vi "Shoot.vi"(3 "Shooter Position (0 to 8)":i8(slide) scale=0.0..4.0) -> (0 "Inside Perimeter":bool=TRUE, 1 "In Position":bool=TRUE)   [LabVIEW 2012]
uses:
  Robot Global Data.vi
  <vilib>/Rock Robotics/WPI/Joystick/WPI_JoystickGetSetRefNum.vi
panel:
  out "Joystick Override":bool=TRUE
  in  "Inbound OLD RBT":dbl=1.7
  in  "Inbound NEW RBT":dbl=1.7
  in  "Upper Perimeter OLD":dbl=0.1
  in  "Lower Perimeter OLD":dbl=3.4
  in  "Rest OLD RBT":dbl=2.5
  in  "Load OLD RBT":dbl=2.5
  in  "Shoot OLD RBT":dbl=1.5
  in  "PID gains\nOLD RBT":T1={"proportional gain (Kc)"=0.5, "integral time (Ti, min)"=0.0, "derivative time (Td, min)"=0.0} {"derivative time (Td, min)" format="%.3f"; "integral time (Ti, min)" format="%.3f"; "proportional gain (Kc)" format="%.3f"}
  in  "Max Speeds\nOLD RBT":cluster{"Down Speed":dbl, "Up Speed":dbl}={"Down Speed"=0.3, "Up Speed"=-0.3} {"Up Speed" format="%.2f"; "Down Speed" format="%.2f"}
  in  "PID gains\nNEW RBT":T1={"proportional gain (Kc)"=0.5, "integral time (Ti, min)"=0.0, "derivative time (Td, min)"=0.0} {"derivative time (Td, min)" format="%.3f"; "integral time (Ti, min)" format="%.3f"; "proportional gain (Kc)" format="%.3f"}
  in  "Max Speeds\nNEW RBT":cluster{"Down Speed":dbl, "Up Speed":dbl}={"Down Speed"=0.2, "Up Speed"=-0.35} {"Up Speed" format="%.2f"; "Down Speed" format="%.2f"}
  in  "Upper Perimeter NEW":dbl=3.8
  in  "Lower Perimeter NEW":dbl=0.6
  in  "Dead Zone":dbl=0.1
  in  "Rest NEW RBT":dbl=4.0
  in  "Load NEW RBT":dbl=0.5
  in  "Shoot NEW RBT":dbl=1.9
  out "output":dbl=0.04258389399999998
  out "Pot Voltage":dbl=0.41483221200000003
  # "OLD"
  # "NEW"
  # "0.5"
  # "0.5"
  # "0.2"
  # "0.3"
  # "0"
  # "0"
  # "-.35"
  # "-0.3"
  # "New"
  # "3"
  # "1.9"
  # "0.6"
  # "2.5"
  # "0.5"
  # "3.8"
  # "2.5"
  # "4"
  # "1.7"
  # "1.7"
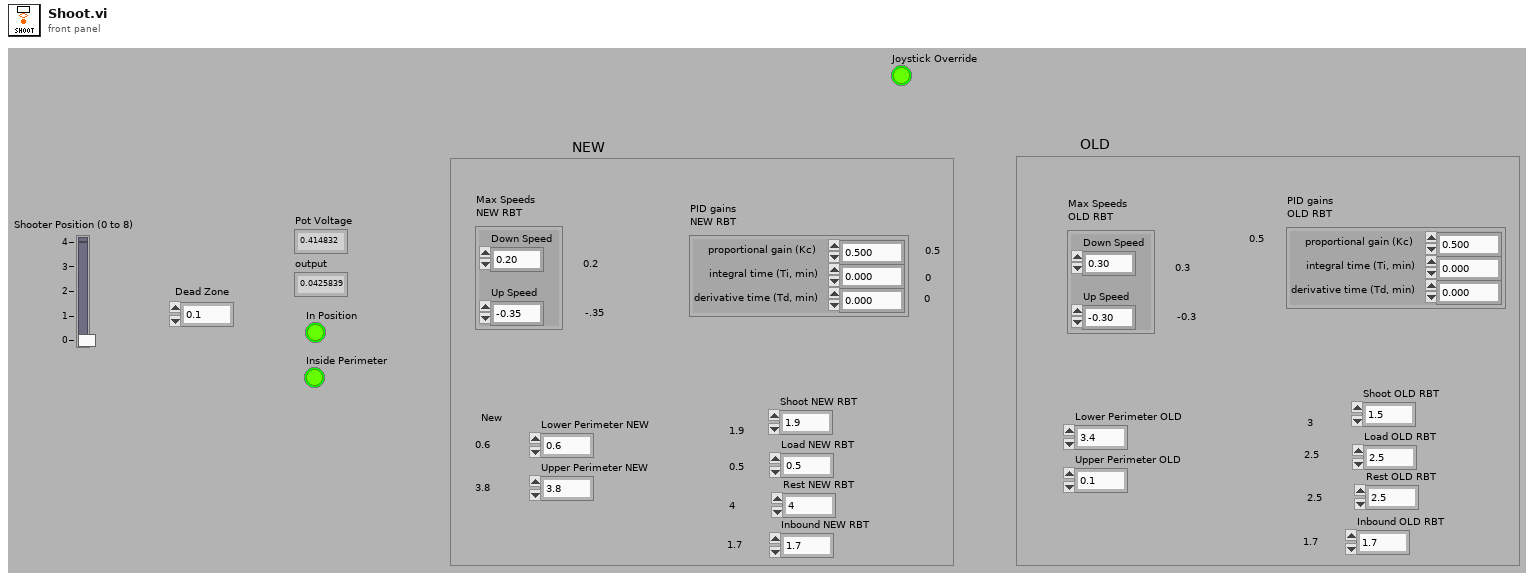
[diagram p1: front panel]
types:
  T1 = cluster{"proportional gain (Kc)":dbl, "integral time (Ti, min)":dbl, "derivative time (Td, min)":dbl}
  T2 = typedef "WPI_JoystickDevRef.ctl" = cluster{"Device":T3}
  T3 = typedef "WPI_JoystickDeviceEnum.ctl" = enum16{"USB 1", "USB 2", "USB 3", "USB 4", "Kinect 1", "Kinect 2"}
  T4 = cluster{"axis 1 (x)":dbl, "axis 2 (y)":dbl, "axis 3 (throttle)":dbl, "axis 4":dbl, "axis 5":dbl, "axis 6":dbl}
  T5 = typedef "WPI_AnalogChannelDevRef.ctl" = cluster{"DevStatus":errorcluster, "Analog Module":T6, "Analog Channel":T7}
  T6 = typedef "FPGA_TypedefAnalogModule.ctl" = enum16{"Analog Module 1", "Analog Module 2"}
  T7 = typedef "FPGA_AIChannel.ctl" = enum8{"AI 1", "AI 2", "AI 3", "AI 4", "AI 5", "AI 6", "AI 7", "AI 8", "Invalid"}
  T8 = typedef "WPI_MotorControlDeviceRef.ctl" = cluster{"DeviceStatus":errorcluster, "Type":enum16{"PWM", "CAN"}, "PWM":cluster{"Digital Module":T9, "PWM Channel":T10, "DeadBand":T11}, "CAN":cluster{"Device Number":u8, "Control Mode":T12, "Semaphore":T13, "Max Vout":dbl}, "Invert":bool, "TransformRef":T14, "InvTransformRef":T14}
  T9 = typedef "FPGA_TypedefDigitalModule.ctl" = enum16{"Digital Module 1", "Digital Module 2"}
  T10 = typedef "FPGA_DIOPWMChannel.ctl" = enum8{"PWM 1", "PWM 2", "PWM 3", "PWM 4", "PWM 5", "PWM 6", "PWM 7", "PWM 8", "PWM 9", "PWM 10", "Invalid"}
  T11 = typedef "WPI_PWMDeadband.ctl" = cluster{"Name":string, "maxPositivePwm":i32, "minPositivePwm":i32, "centerPwm":i32, "maxNegativePwm":i32, "minNegativePwm":i32, "angularRange":u16}
  T12 = typedef "WPI_CANJaguar_ControlMode.ctl" = enum8{"Percent VBus", "Current", "Speed", "Position", "Voltage"}
  T13 = typedef "Semaphore RefNum" = refnum<k1>
  T14 = typedef "WPI_PWMTransform_ConPane.ctl" = refnum<vi>
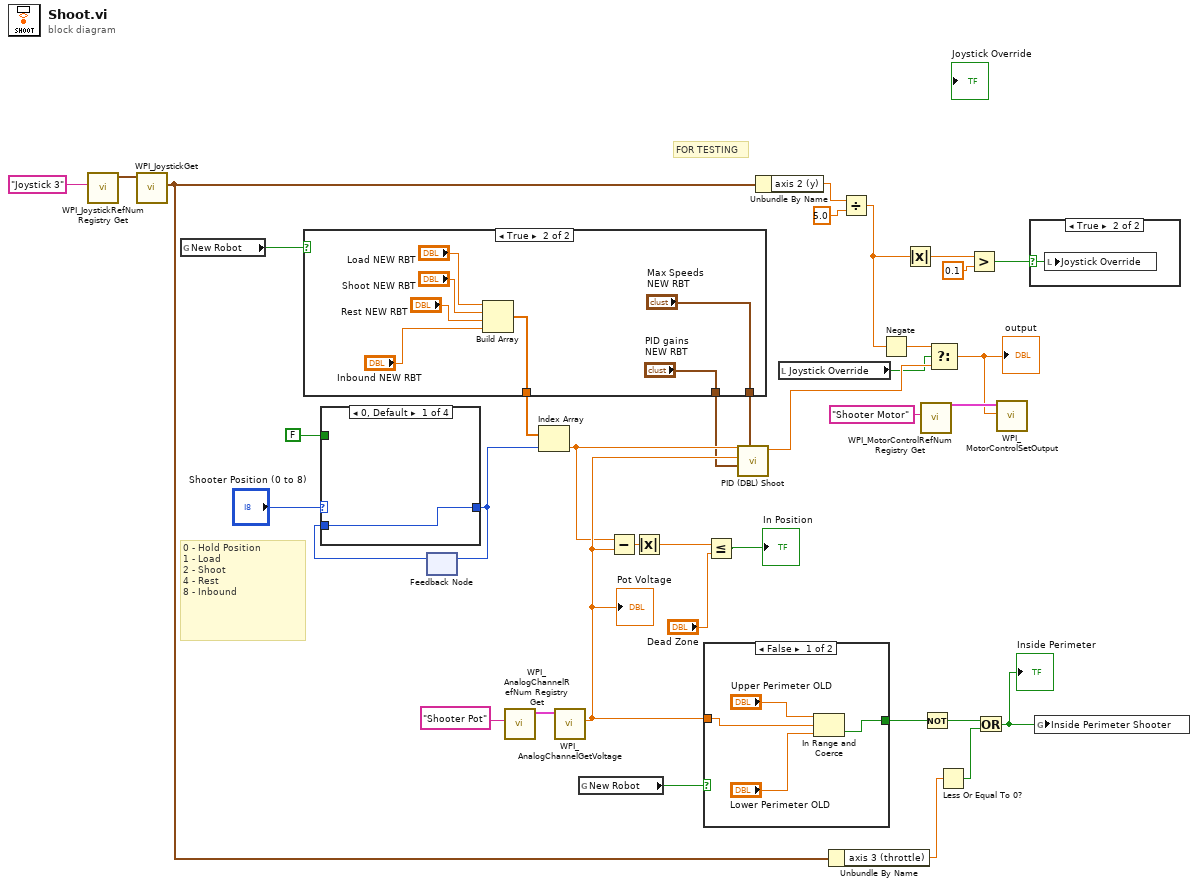
[diagram p0: block diagram]
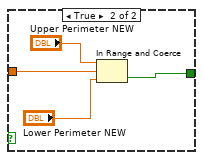
[diagram p3: hidden frame]
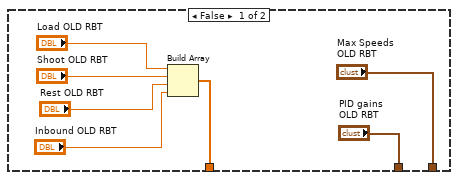
[diagram p4: hidden frame]
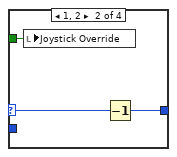
[diagram p5: hidden frame]
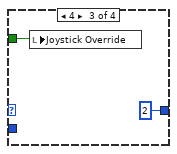
[diagram p6: hidden frame]
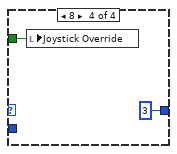
[diagram p7: hidden frame]
diagram:
  # "FOR TESTING"
  # "0 - Hold Position\n1 - Load\n2 - Shoot\n4 - Rest\n8 - Inbound"
  n1 = call <vilib>:"WPI_JoystickRefNum Registry Get.vi"("refnum name"="Joystick 3") -> ("JoystickDevRef"=w14:T2)  [unwired: 9 in, 1 out]
  n2 = call <vilib>:"WPI_JoystickGet.vi"("JoystickDevRef"=w14) -> ("Axes"=w6:T4)  [unwired: 4 in, 2 out]
  n3 = global read "Robot Global Data.vi" "New Robot"() -> (w20:bool)
  n4 = case shown="True" w20 {
    tunnel: [w42 w50] -> w33
    tunnel: ["Max Speeds\nOLD RBT" "Max Speeds\nNEW RBT"] -> w25
    tunnel: ["PID gains\nOLD RBT" "PID gains\nNEW RBT"] -> w22
    frame False {
      n5 = Build Array("Load OLD RBT", "Shoot OLD RBT", "Rest OLD RBT", "Inbound OLD RBT") -> (w42:dbl[])
    }
    frame True {
      n6 = Build Array("Load NEW RBT", "Shoot NEW RBT", "Rest NEW RBT", "Inbound NEW RBT") -> (w50:dbl[])
    }
  }
  n7 = feedback #1() -> (w28:i8)  [unwired: 1 in]
  n8 = case shown="0, Default" "Shooter Position (0 to 8)" {
    selector: "Shooter Position (0 to 8)" -> [_ w55 _ _]
    tunnel: w28 -> [w52 _ _ _]
    tunnel: [w52 w54 i8 2 i8 3] -> w27
    tunnel: FALSE -> [_ w53 w56 w58]
    frame 0, Default {
    }
    frame 1, 2 {
      n9 = local write "Joystick Override"(w53) -> ()
      n10 = Decrement(x=w55) -> (x-1=w54:i8)
    }
    frame 4 {
      n11 = local write "Joystick Override"(w56) -> ()
    }
    frame 8 {
      n12 = local write "Joystick Override"(w58) -> ()
    }
  }
  n13 = feedback-in #1(w27) -> ()
  n14 = call <vilib>:"WPI_AnalogChannelRefNum Registry Get.vi"("refnum name"="Shooter Pot") -> ("AIDeviceRef"=w35:T5)  [unwired: 9 in, 1 out]
  n15 = Index Array(array=w33, index=w27) -> (element=w23:dbl)
  n16 = call <vilib>:"WPI_AnalogChannelGetVoltage.vi"("AIDeviceRef"=w35) -> ("Voltage"=w24:dbl)  [unwired: 8 in, 2 out]
  "Pot Voltage" <- w24
  n17 = global read "Robot Global Data.vi" "New Robot"() -> (w21:bool)
  n18 = Subtract(x=w23, y=w24) -> (x-y=w32:dbl)
  n19 = Absolute Value(x=w32) -> (abs(x)=w31:dbl)
  n20 = case shown="False" w21 {
    tunnel: [w63 w67] -> w26
    tunnel: w24 -> [w62 w64]
    frame False {
      n21 = In Range and Coerce(upper limit="Upper Perimeter OLD", x=w62, lower limit="Lower Perimeter OLD") -> (In Range?=w63:bool)  [unwired: 1 out]
    }
    frame True {
      n22 = In Range and Coerce(upper limit="Upper Perimeter NEW", x=w64, lower limit="Lower Perimeter NEW") -> (In Range?=w67:bool)  [unwired: 1 out]
    }
  }
  n23 = Less Or Equal?(x=w31, y="Dead Zone") -> (x <= y?=→"In Position":bool)
  n24 = call "PID (DBL) Shoot.vi"("output range"=w25, "PID gains"=w22, "process variable"=w24, "setpoint"=w23) -> ("output"=w17:dbl)  [unwired: 6 in, 1 out]
  n25 = Unbundle By Name(w6) -> ("axis 2 (y)"=w10:dbl)
  n26 = local read "Joystick Override"() -> (w3:bool)
  n27 = Unbundle By Name(w6) -> ("axis 3 (throttle)"=w9:dbl)
  n28 = Divide(x=w10, y=5.0) -> (x/y=w12:dbl)
  n29 = Negate(x=w12) -> (-x=w4:dbl)
  n30 = Absolute Value(x=w12) -> (abs(x)=w18:dbl)
  n31 = call <vilib>:"WPI_MotorControlRefNum Registry Get.vi"("refnum name"="Shooter Motor") -> ("MotorControlDevRef"=w37:T8)  [unwired: 9 in, 1 out]
  n32 = Not(x=w26) -> (.not. x?=w5:bool)
  n33 = Select(t=w4, s=w3, f=w17) -> (s? t:f=w16:dbl)
  "output" <- w16
  n34 = Less Or Equal To 0?(x=w9) -> (x <= 0?=w8:bool)
  n35 = Greater?(x=w18, y=0.1) -> (0:w2:bool)
  n36 = Or(x=w5, y=w8) -> (x .or. y?=w7:bool)
  "Inside Perimeter" <- w7
  n37 = call <vilib>:"WPI_MotorControlSetOutput.vi"("Output"=w16, "MotorControlDevRef"=w37) -> ()  [unwired: 7 in, 3 out]
  n38 = case shown="True" w2 {
    selector: w2 -> [_ w68]
    frame False {
    }
    frame True {
      n39 = local write "Joystick Override"(w68) -> ()
    }
  }
  n40 = global write "Robot Global Data.vi" "Inside Perimeter Shooter"(w7) -> ()
